vi "FeedbackDecode_DEKASensorsRaw2Real.vi"(1 "SensorsRaw":T1={"x241"=[0, 0, 0, 0, 0, 0, 0, 0], "x341"=[0, 0, 0, 0, 0, 0, 0, 0], "x4C2"=[0, 0, 0, 0, 0, 0, 0, 0], "x4AA"=[0, 0, 0, 0, 0, 0, 0, 0], "x4BF"=[0, 0, 0, 0, 0, 0, 0, 0]}, 2 "Calibration?":bool) -> (0 "Sensors":T2)   [LabVIEW 2020]
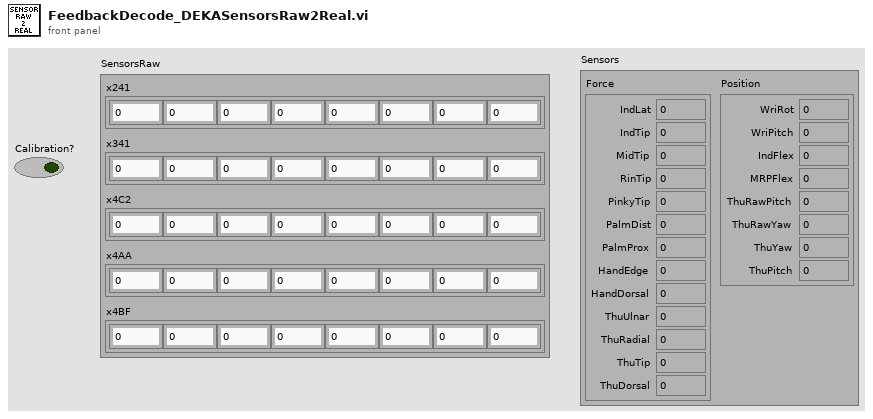
[diagram p1: front panel]
types:
  T1 = cluster{"x241":u8[], "x341":u8[], "x4C2":u8[], "x4AA":u8[], "x4BF":u8[]}
  T2 = cluster{"Position":cluster{"WriRot":dbl, "WriPitch":dbl, "IndFlex":dbl, "MRPFlex":dbl, "ThuRawPitch":dbl, "ThuRawYaw":dbl, "ThuYaw":dbl, "ThuPitch":dbl}, "Force":cluster{"IndLat":dbl, "IndTip":dbl, "MidTip":dbl, "RinTip":dbl, "PinkyTip":dbl, "PalmDist":dbl, "PalmProx":dbl, "HandEdge":dbl, "HandDorsal":dbl, "ThuUlnar":dbl, "ThuRadial":dbl, "ThuTip":dbl, "ThuDorsal":dbl}}
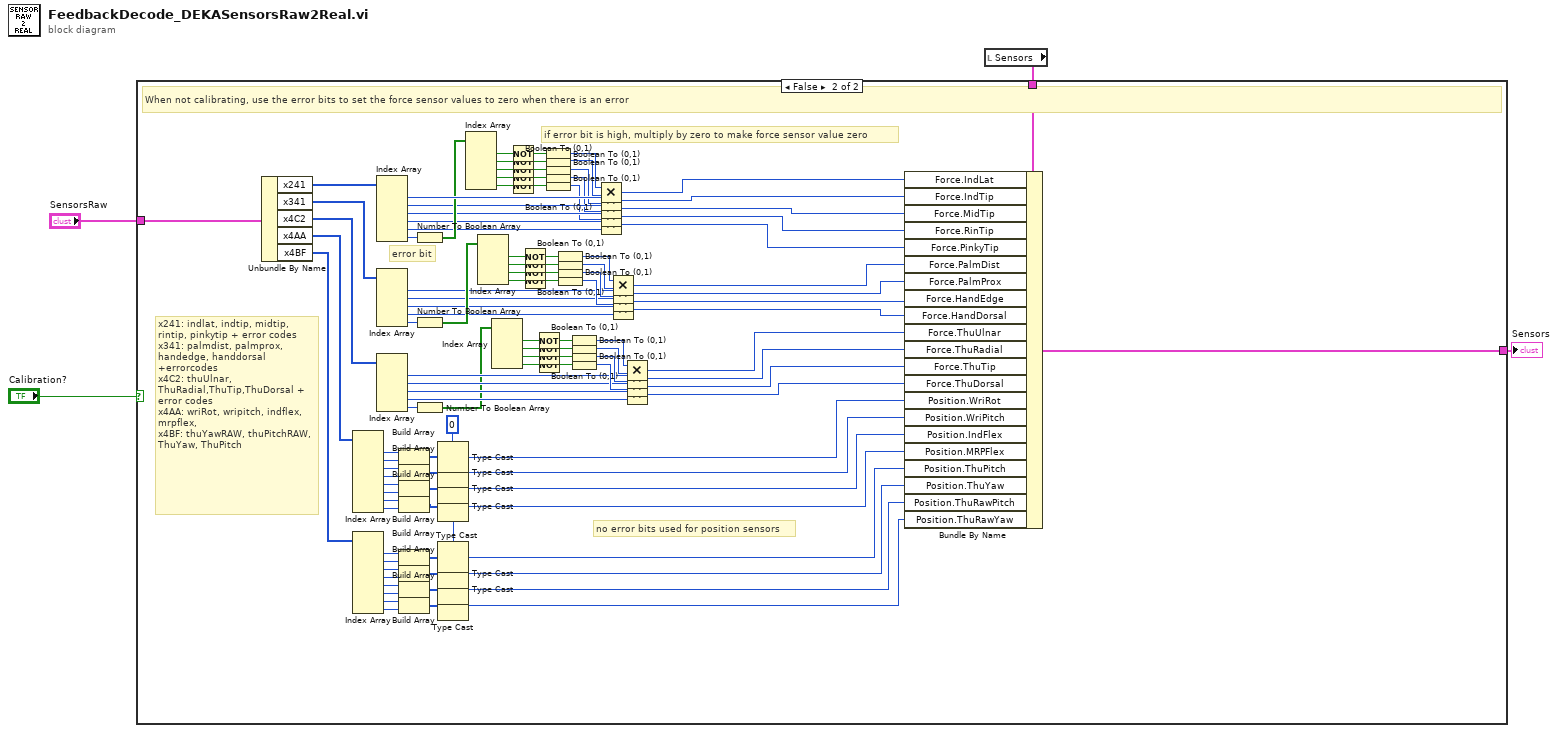
[diagram p0: block diagram]
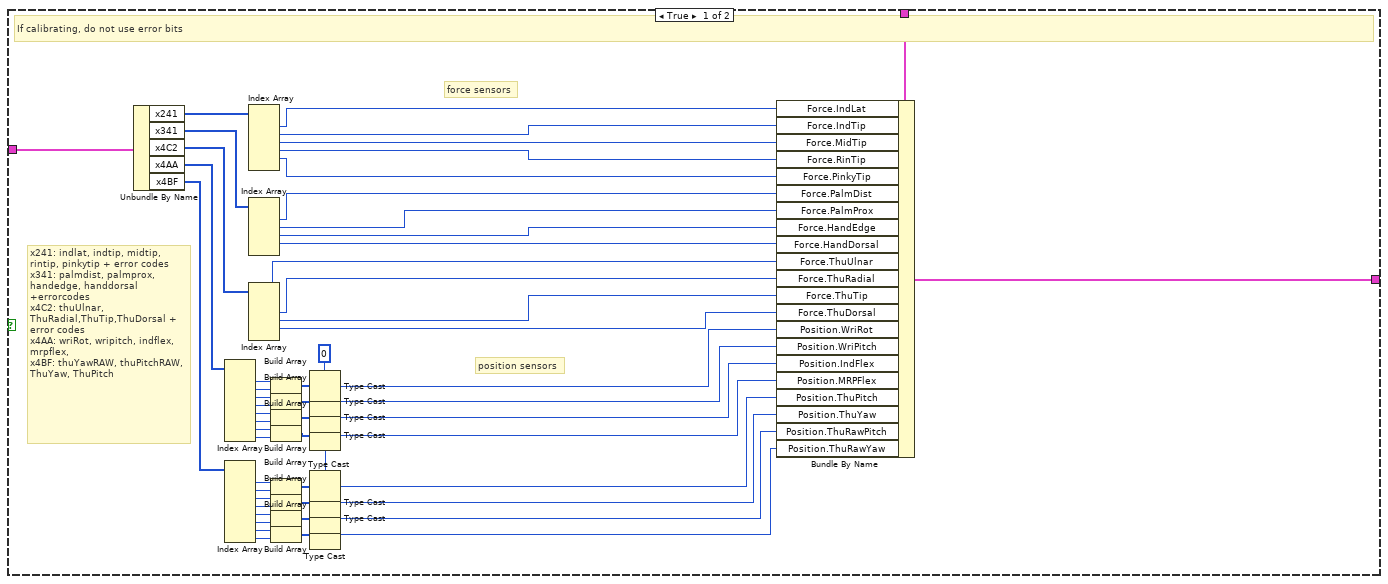
[diagram p2: hidden frame]
diagram:
  n1 = local read "Sensors"() -> (w4:T2)
  n2 = case shown="False" "Calibration?" {
    tunnel: w4 -> [w21 w133]
    tunnel: "SensorsRaw" -> [w7 w61]
    tunnel: [w6 w60] -> w2
    frame True {
      w23 = i16 0
      # "position sensors"
      # "force sensors"
      # "x241: indlat, indtip, midtip, rintip, pinkytip + error codes\nx341: palmdist, palmprox, handedge, handdorsal +errorcodes\nx4C2: thuUlnar, ThuRadial,ThuTip,ThuDorsal + error codes\nx4AA: wriRot, wripitch, indflex, mrpflex,\nx4BF: thuYawRAW, thuPitchRAW, ThuYaw, ThuPitch"
      # "If calibrating, do not use error bits"
      n3 = Unbundle By Name(w7) -> ("x241"=w58:u8[], "x341"=w57:u8[], "x4C2"=w56:u8[], "x4AA"=w55:u8[], "x4BF"=w34:u8[])
      n4 = Index Array(array=w55) -> (element #1=w54:u8, element #2=w53:u8, element #3=w50:u8, element #4=w49:u8, element #5=w46:u8, element #6=w45:u8, element #7=w42:u8, element #8=w41:u8)  [unwired: 8 in]
      n5 = Index Array(array=w34) -> (element #1=w36:u8, element #2=w35:u8, element #3=w30:u8, element #4=w29:u8, element #5=w27:u8, element #6=w26:u8, element #7=w24:u8, element #8=w5:u8)  [unwired: 8 in]
      n6 = Index Array(array=w58) -> (element #1=w20:u8, element #2=w19:u8, element #3=w18:u8, element #4=w17:u8, element #5=w16:u8)  [unwired: 6 in, 1 out]
      n7 = Index Array(array=w57) -> (element #1=w15:u8, element #2=w14:u8, element #3=w13:u8, element #4=w12:u8)  [unwired: 5 in, 1 out]
      n8 = Index Array(array=w56) -> (element #1=w11:u8, element #2=w10:u8, element #3=w9:u8, element #4=w8:u8)  [unwired: 5 in, 1 out]
      n9 = Build Array(w54, w53) -> (w52:u8[])
      n10 = Build Array(w50, w49) -> (w48:u8[])
      n11 = Build Array(w46, w45) -> (w44:u8[])
      n12 = Build Array(w42, w41) -> (w40:u8[])
      n13 = Build Array(w36, w35) -> (w38:u8[])
      n14 = Build Array(w30, w29) -> (w33:u8[])
      n15 = Build Array(w27, w26) -> (w32:u8[])
      n16 = Build Array(w24, w5) -> (w31:u8[])
      n17 = Type Cast(type=w23, x=w52) -> (*(type *) &x=w51:i16)
      n18 = Type Cast(type=w23, x=w48) -> (*(type *) &x=w47:i16)
      n19 = Type Cast(type=w23, x=w44) -> (*(type *) &x=w43:i16)
      n20 = Type Cast(type=w23, x=w40) -> (*(type *) &x=w39:i16)
      n21 = Type Cast(type=w23, x=w38) -> (*(type *) &x=w37:i16)
      n22 = Type Cast(type=w23, x=w33) -> (*(type *) &x=w28:i16)
      n23 = Type Cast(type=w23, x=w32) -> (*(type *) &x=w25:i16)
      n24 = Type Cast(type=w23, x=w31) -> (*(type *) &x=w22:i16)
      n25 = Bundle By Name(cluster=w21, "Force.IndLat"=w20, "Force.IndTip"=w19, "Force.MidTip"=w18, "Force.RinTip"=w17, "Force.PinkyTip"=w16, "Force.PalmDist"=w15, "Force.PalmProx"=w14, "Force.HandEdge"=w13, "Force.HandDorsal"=w12, "Force.ThuUlnar"=w11, "Force.ThuRadial"=w10, "Force.ThuTip"=w9, "Force.ThuDorsal"=w8, "Position.WriRot"=w51, "Position.WriPitch"=w47, "Position.IndFlex"=w43, "Position.MRPFlex"=w39, "Position.ThuPitch"=w37, "Position.ThuYaw"=w28, "Position.ThuRawPitch"=w25, "Position.ThuRawYaw"=w22) -> (w6:T2)
    }
    frame False {
      w135 = i16 0
      # "no error bits used for position sensors"
      # "if error bit is high, multiply by zero to make force sensor value zero"
      # "error bit"
      # "x241: indlat, indtip, midtip, rintip, pinkytip + error codes\nx341: palmdist, palmprox, handedge, handdorsal +errorcodes\nx4C2: thuUlnar, ThuRadial,ThuTip,ThuDorsal + error codes\nx4AA: wriRot, wripitch, indflex, mrpflex,\nx4BF: thuYawRAW, thuPitchRAW, ThuYaw, ThuPitch"
      # "When not calibrating, use the error bits to set the force sensor values to zero when there is an error"
      n26 = Unbundle By Name(w61) -> ("x241"=w170:u8[], "x341"=w169:u8[], "x4C2"=w168:u8[], "x4AA"=w167:u8[], "x4BF"=w146:u8[])
      n27 = Index Array(array=w167) -> (element #1=w166:u8, element #2=w165:u8, element #3=w162:u8, element #4=w161:u8, element #5=w158:u8, element #6=w157:u8, element #7=w154:u8, element #8=w153:u8)  [unwired: 8 in]
      n28 = Index Array(array=w146) -> (element #1=w148:u8, element #2=w147:u8, element #3=w142:u8, element #4=w141:u8, element #5=w139:u8, element #6=w138:u8, element #7=w136:u8, element #8=w59:u8)  [unwired: 8 in]
      n29 = Index Array(array=w170) -> (element #1=w131:u8, element #2=w126:u8, element #3=w125:u8, element #4=w124:u8, element #5=w123:u8, element #6=w132:u8)  [unwired: 6 in]
      n30 = Index Array(array=w169) -> (element #1=w93:u8, element #2=w92:u8, element #3=w91:u8, element #4=w90:u8, element #5=w89:u8)  [unwired: 5 in]
      n31 = Index Array(array=w168) -> (element #1=w75:u8, element #2=w74:u8, element #3=w73:u8, element #4=w72:u8, element #5=w71:u8)  [unwired: 5 in]
      n32 = Build Array(w166, w165) -> (w164:u8[])
      n33 = Build Array(w162, w161) -> (w160:u8[])
      n34 = Build Array(w158, w157) -> (w156:u8[])
      n35 = Build Array(w154, w153) -> (w152:u8[])
      n36 = Build Array(w148, w147) -> (w150:u8[])
      n37 = Build Array(w142, w141) -> (w145:u8[])
      n38 = Build Array(w139, w138) -> (w144:u8[])
      n39 = Build Array(w136, w59) -> (w143:u8[])
      n40 = Number To Boolean Array(number=w132) -> (Boolean array=w130:bool[])
      n41 = Number To Boolean Array(number=w89) -> (Boolean array=w94:bool[])
      n42 = Number To Boolean Array(number=w71) -> (Boolean array=w70:bool[])
      n43 = Type Cast(type=w135, x=w164) -> (*(type *) &x=w163:i16)
      n44 = Type Cast(type=w135, x=w160) -> (*(type *) &x=w159:i16)
      n45 = Type Cast(type=w135, x=w156) -> (*(type *) &x=w155:i16)
      n46 = Type Cast(type=w135, x=w152) -> (*(type *) &x=w151:i16)
      n47 = Type Cast(type=w135, x=w150) -> (*(type *) &x=w149:i16)
      n48 = Type Cast(type=w135, x=w145) -> (*(type *) &x=w140:i16)
      n49 = Type Cast(type=w135, x=w144) -> (*(type *) &x=w137:i16)
      n50 = Type Cast(type=w135, x=w143) -> (*(type *) &x=w134:i16)
      n51 = Index Array(array=w130) -> (element #1=w128:bool, element #2=w113:bool, element #3=w112:bool, element #4=w111:bool, element #5=w110:bool)  [unwired: 5 in]
      n52 = Index Array(array=w94) -> (element #1=w96:bool, element #2=w101:bool, element #3=w102:bool, element #4=w103:bool)  [unwired: 4 in]
      n53 = Index Array(array=w70) -> (element #1=w69:bool, element #2=w81:bool, element #3=w80:bool, element #4=w79:bool)  [unwired: 4 in]
      n54 = Not(x=w128) -> (.not. x?=w129:bool)
      n55 = Not(x=w113) -> (.not. x?=w117:bool)
      n56 = Not(x=w112) -> (.not. x?=w116:bool)
      n57 = Not(x=w111) -> (.not. x?=w115:bool)
      n58 = Not(x=w110) -> (.not. x?=w114:bool)
      n59 = Not(x=w96) -> (.not. x?=w95:bool)
      n60 = Not(x=w101) -> (.not. x?=w98:bool)
      n61 = Not(x=w102) -> (.not. x?=w99:bool)
      n62 = Not(x=w103) -> (.not. x?=w100:bool)
      n63 = Not(x=w69) -> (.not. x?=w68:bool)
      n64 = Not(x=w81) -> (.not. x?=w84:bool)
      n65 = Not(x=w80) -> (.not. x?=w83:bool)
      n66 = Not(x=w79) -> (.not. x?=w82:bool)
      n67 = Boolean To (0,1)(Boolean=w129) -> (0, 1=w122:i16)
      n68 = Boolean To (0,1)(Boolean=w117) -> (0, 1=w62:i16)
      n69 = Boolean To (0,1)(Boolean=w116) -> (0, 1=w109:i16)
      n70 = Boolean To (0,1)(Boolean=w115) -> (0, 1=w108:i16)
      n71 = Boolean To (0,1)(Boolean=w114) -> (0, 1=w107:i16)
      n72 = Boolean To (0,1)(Boolean=w95) -> (0, 1=w97:i16)
      n73 = Boolean To (0,1)(Boolean=w98) -> (0, 1=w104:i16)
      n74 = Boolean To (0,1)(Boolean=w99) -> (0, 1=w105:i16)
      n75 = Boolean To (0,1)(Boolean=w100) -> (0, 1=w106:i16)
      n76 = Boolean To (0,1)(Boolean=w68) -> (0, 1=w67:i16)
      n77 = Boolean To (0,1)(Boolean=w84) -> (0, 1=w78:i16)
      n78 = Boolean To (0,1)(Boolean=w83) -> (0, 1=w77:i16)
      n79 = Boolean To (0,1)(Boolean=w82) -> (0, 1=w76:i16)
      n80 = Multiply(x=w122, y=w131) -> (x*y=w127:i16)
      n81 = Multiply(x=w62, y=w126) -> (x*y=w121:i16)
      n82 = Multiply(x=w109, y=w125) -> (x*y=w120:i16)
      n83 = Multiply(x=w108, y=w124) -> (x*y=w119:i16)
      n84 = Multiply(x=w107, y=w123) -> (x*y=w118:i16)
      n85 = Multiply(x=w97, y=w93) -> (x*y=w88:i16)
      n86 = Multiply(x=w104, y=w92) -> (x*y=w87:i16)
      n87 = Multiply(x=w105, y=w91) -> (x*y=w86:i16)
      n88 = Multiply(x=w106, y=w90) -> (x*y=w85:i16)
      n89 = Multiply(x=w67, y=w75) -> (x*y=w66:i16)
      n90 = Multiply(x=w78, y=w74) -> (x*y=w65:i16)
      n91 = Multiply(x=w77, y=w73) -> (x*y=w64:i16)
      n92 = Multiply(x=w76, y=w72) -> (x*y=w63:i16)
      n93 = Bundle By Name(cluster=w133, "Force.IndLat"=w127, "Force.IndTip"=w121, "Force.MidTip"=w120, "Force.RinTip"=w119, "Force.PinkyTip"=w118, "Force.PalmDist"=w88, "Force.PalmProx"=w87, "Force.HandEdge"=w86, "Force.HandDorsal"=w85, "Force.ThuUlnar"=w66, "Force.ThuRadial"=w65, "Force.ThuTip"=w64, "Force.ThuDorsal"=w63, "Position.WriRot"=w163, "Position.WriPitch"=w159, "Position.IndFlex"=w155, "Position.MRPFlex"=w151, "Position.ThuPitch"=w149, "Position.ThuYaw"=w140, "Position.ThuRawPitch"=w137, "Position.ThuRawYaw"=w134) -> (w60:T2)
    }
  }
  "Sensors" <- w2
